vi "Scanned Read - Input Module.vi"(6 "Model":T1, 7 "Channel Type":T3, 8 "error in (no error)":errorcluster, 9 "IOV ref":refnum<k21>, 11 "IOV ref in":T2) -> (0 "error out":errorcluster, 1 "channel data":dbl[](array[numeric]), 3 "IOV ref out":T2)   [LabVIEW 2011, in "Scan Engine Custom Device.lvlib"]
uses:
  Scan Engine Custom Device.lvlib
  Modules.lvlibp/RSI Module/Channel Type.ctl
  Type Defs/Open Module IOVs.ctl
  Modules.lvlibp/RSI Module/Module Models.ctl
  Modules.lvlibp/RSI Module/RSI Module.lvclass
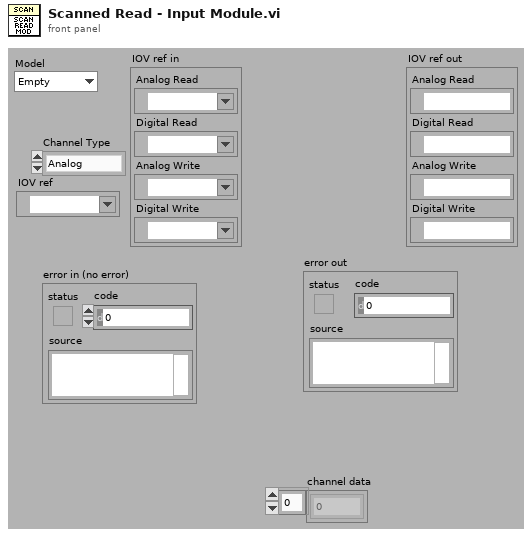
[diagram p1: front panel]
types:
  T1 = typedef "Modules.lvlibp/RSI Module.lvclass/Module Models.ctl" = enum16{"Empty", "NI 9201", "NI 9203", "NI 9205", "NI 9206", "NI 9207", "NI 9208", "NI 9211", "NI 9213", "NI 9214", "NI 9215", "NI 9217", "NI 9219", "NI 9221", "NI 9225", "NI 9227", "NI 9229", "NI 9233", "NI 9234", "NI 9235", "NI 9236", "NI 9237", "NI 9239", "NI 9263", "NI 9264", "NI 9265", "NI 9269", "NI 9375", "NI 9401", "NI 9402", "NI 9403", "NI 9411", "NI 9421", "NI 9422", "NI 9423", "NI 9425", "NI 9426", "NI 9435", "NI 9472", "NI 9474", "NI 9475", "NI 9476", "NI 9477", "NI 9478", "NI 9481", "NI 9482", "NI 9485"}
  T2 = typedef "Scan Engine Custom Device.lvlib/Open Module IOVs.ctl" = cluster{"Analog Read":refnum<k21>, "Digital Read":refnum<k21>, "Analog Write":refnum<k21>, "Digital Write":refnum<k21>}
  T3 = typedef "Modules.lvlibp/RSI Module.lvclass/Channel Type.ctl" = enum16{"Analog", "Digital"}
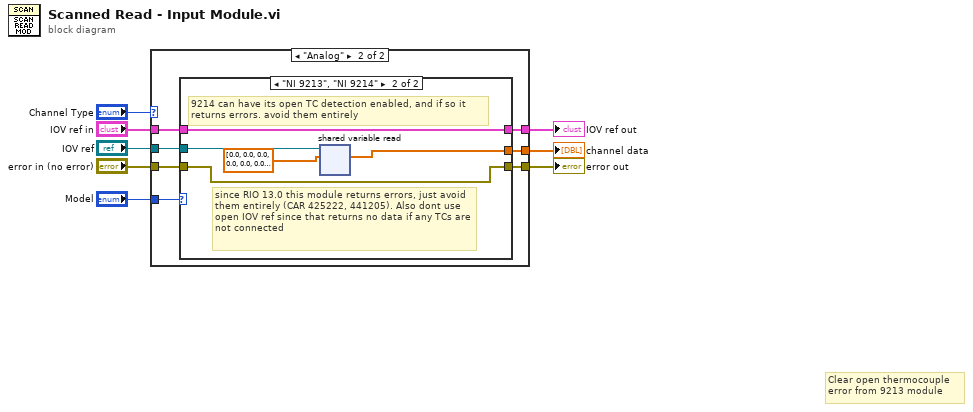
[diagram p0: block diagram]
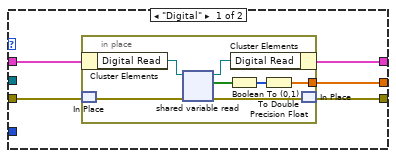
[diagram p2: hidden frame]
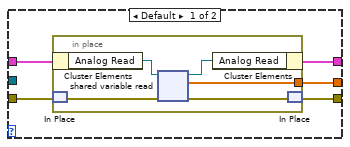
[diagram p3: hidden frame]
diagram:
  # "Clear open thermocouple\nerror from 9213 module"
  n1 = case shown="\"Analog\"" "Channel Type" {
    tunnel: "IOV ref in" -> [w13 w27]
    tunnel: "error in (no error)" -> [w9 w25]
    tunnel: [w10 w24] -> w4
    tunnel: [w12 w26] -> w5
    tunnel: [w11 w23] -> w3
    tunnel: "Model" -> [_ w22]
    tunnel: "IOV ref" -> [_ w21]
    frame "Digital" {
      n2 = in-place {
        in-place-border: [w17] -> w11
        n3 = in-place-cluster #1(w13) -> ("Digital Read"=w20:refnum<k21>)
        n4 = in-place-match #2(w9) -> (w14:errorcluster)
        n5 = shared-variable-read(w20, w14) -> (w19:refnum<k21>, w15:errorcluster, w16:bool[])
        n6 = Boolean To (0,1)(Boolean=w16) -> (0, 1=w18:i16[])
        n7 = in-place-cluster #1("Digital Read"=w19) -> (w12:T2)
        n8 = To Double Precision Float(number=w18) -> (double precision float=w17:dbl[])
        n9 = in-place-match #2(w15) -> (w10:errorcluster)
      }
    }
    frame "Analog" {
      n10 = case shown="\"NI 9213\", \"NI 9214\"" w22 {
        tunnel: w27 -> [w32 w41]
        tunnel: [w31 w41] -> w26
        tunnel: w25 -> [w29 w42]
        tunnel: [w28 w42] -> w24
        tunnel: [w30 w38] -> w23
        tunnel: w21 -> [_ w40]
        frame Default {
          n11 = in-place {
            in-place-border: [w35] -> w30
            n12 = in-place-cluster #3(w32) -> ("Analog Read"=w37:refnum<k21>)
            n13 = in-place-match #4(w29) -> (w34:errorcluster)
            n14 = shared-variable-read(w37, w34) -> (w36:refnum<k21>, w33:errorcluster, w35:dbl[])
            n15 = in-place-cluster #3("Analog Read"=w36) -> (w31:T2)
            n16 = in-place-match #4(w33) -> (w28:errorcluster)
          }
        }
        frame "NI 9213", "NI 9214" {
          # "9214 can have its open TC detection enabled, and if so it returns errors. avoid them entirely"
          # "since RIO 13.0 this module returns errors, just avoid them entirely (CAR 425222, 441205). Also dont use open IOV ref since that returns no data if any TCs are not connected"
          n17 = shared-variable-read(w40, dbl[] [0.0, 0.0, 0.0, 0.0, 0.0, 0.0, 0.0, 0.0, 0.0, 0.0, 0.0, 0.0, 0.0, 0.0, 0.0, 0.0]) -> (w38:dbl[])  [unwired: 1 in, 2 out]
        }
      }
    }
  }
  "error out" <- w4
  "channel data" <- w3
  "IOV ref out" <- w5
